vi "OpenDB.vi"(8 "Error In":errorcluster, 9 "Password":string, 10 "Username":string, 11 "DB-Name":string) -> (0 "Error Out":errorcluster, 3 "DBref":T1)   [LabVIEW 2017, in "Server.lvlib" / "Oracle.lvlib"]
uses:
  Oracle.lvlib
  <vilib>/addons/database/Connection.llb/Conn ObjectReference.ctl
  <vilib>/addons/database/Connection.llb/DB Tools Open Connec (String).vi
  <vilib>/addons/database/NI_Database_API.lvlib
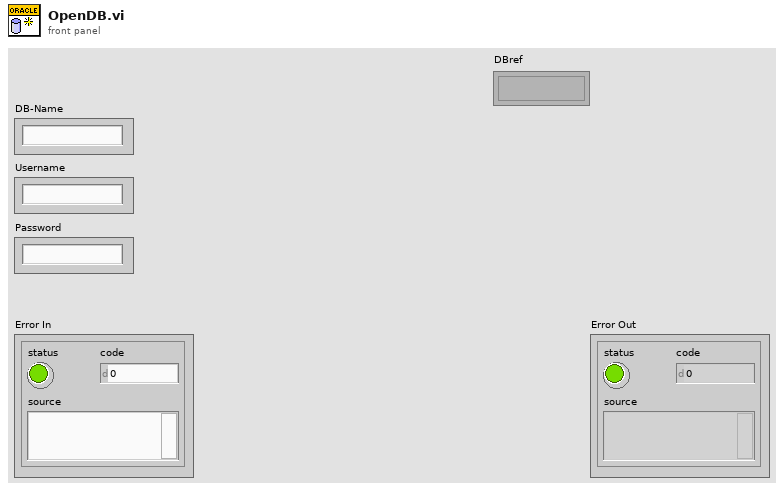
[diagram p1: front panel]
types:
  T1 = typedef "NI_Database_API.lvlib/Conn ObjectReference.ctl" = refnum<k1>
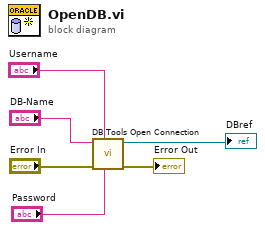
[diagram p0: block diagram]
diagram:
  n1 = call-poly <vilib>:"DB Tools Open Connection.vi"("password"="Password", "userID"="Username", "error in (no error)"="Error In", "connection information"="DB-Name") -> ("error out"=→"Error Out":errorcluster, "connection reference"=→"DBref":T1)  [unwired: 4 in]
